vi "Initialize TS Engine.vi"(8 "error in (no error)":errorcluster, 11 "niRFSTS Sequence Flow in":refnum<class "niRFSTS Sequence Flow.lvclass">) -> (0 "error out":errorcluster, 3 "niRFSTS Sequence Flow out":refnum<class "niRFSTS Sequence Flow.lvclass">)   [LabVIEW 2018, in "niRFSTS Sequence Flow.lvclass"]
uses:
  niRFSTS Sequence Flow.lvclass
  niRFSTS Sequence Flow.lvclass/niRFSTS Sequence Flow.ctl
  Plugins/TestStand API Tools (TSAT).lvlibp/TSAT Engine Actions/TSAT Engine Actions.lvlib
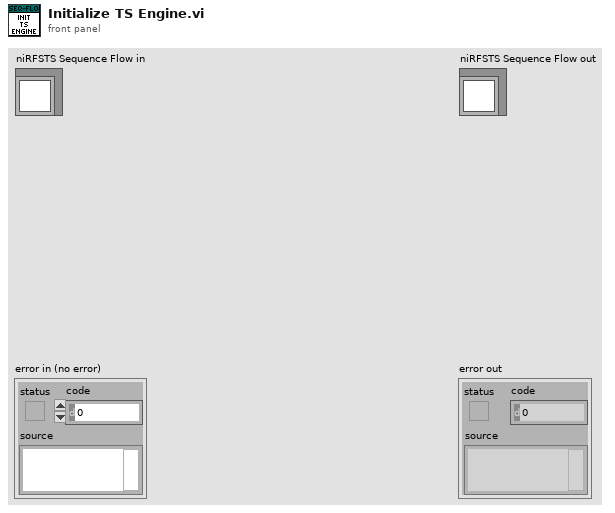
[diagram p1: front panel]
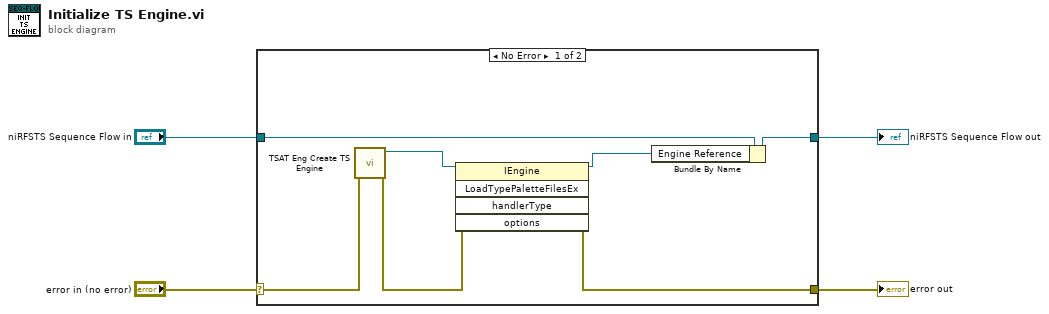
[diagram p0: block diagram]
diagram:
  n1 = case shown="No Error" "error in (no error)" {
    selector: "error in (no error)" -> [w8 w13]
    tunnel: [w5 w13] -> w3
    tunnel: [w7 w12] -> w1
    tunnel: "niRFSTS Sequence Flow in" -> [w11 w12]
    frame No Error {
      n2 = call "TSAT Eng Create TS Engine.vi"("Error In"=w8) -> ("Error out"=w10:errorcluster, "Engine Reference"=w9:refnum<k7>)  [unwired: 9 in]
      n3 = invoke class="IEngine" method="LoadTypePaletteFilesEx"(reference=w9, error in=w10) -> (reference out=w6:refnum<k7>, error out=w5:errorcluster)  [unwired: 3 in, 3 out]
      n4 = Bundle By Name(cluster=w11, "Engine Reference"=w6) -> (w7:refnum<class "niRFSTS Sequence Flow.lvclass">)
    }
    frame Error {
    }
  }
  "error out" <- w3
  "niRFSTS Sequence Flow out" <- w1
